vi "Get All Errors Arrays.vi"() -> (0 "All Error Codes out":i32[](array[numeric]), 1 "All Error Messages out":string[](array[string]), 2 "All Errors Criticality out":i32[](array[numeric]))   [LabVIEW 2026, in "TALOS.lvlib" / "Error Memory.lvlib"]
uses:
  Error Memory.lvlib
  Error Memory Core Enum.ctl
  Support VIs/Circus Root Path.vi
  Error Crt Lvl checker.vi
  Error Memory Core.vi/40c8088d-b597-4017-91af-faa98e00292e.vi
  Error Memory Core.vi/d4a3ab98-063c-4e44-b43d-fbdcfe6c2be2.vi
  Support VIs/Is in Packed Library.vi
  Support VIs/TALOS Root path.vi
  Support VIs/Read CSV worksheet.vi
  Support VIs/Global Memory.vi
  Support VIs/Global Constants.vi
  <vilib>/Comparison/Equal/Equal Functor/Equal Functor.lvclass
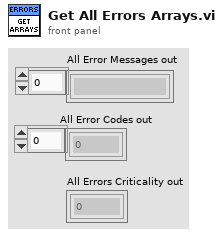
[diagram p1: front panel]
types:
  T1 = typedef "TALOS.lvlib/Error Memory.lvlib/Error Memory Core Enum.ctl" = enum16{"Init", "Get Error Message from Code", "Get All Errors", "Get Error Criticality from Code"}
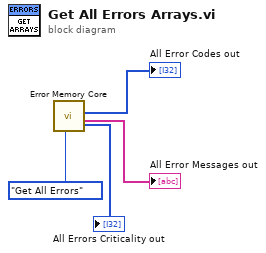
[diagram p0: block diagram]
diagram:
  n1 = call "Error Memory Core.vi"("Error Memory Core Enum"=Error_Memory_Core_Enum."Get All Errors") -> ("All Error Messages out"=→"All Error Messages out":string[], "All Error Codes out"=→"All Error Codes out":i32[], "All Errors Criticality out"=→"All Errors Criticality out":u8[])  [unwired: 5 in, 3 out]
